vi "Webcam - Obstacle Box.vi"(0 "Image In":T1, 1 "Font, Size & Style":T2={"Desired Font (Application)"=enum."User-specified Font", "[User-specified Font]"={"Font Name"="", "Size"=50, "Strikeout?"=FALSE, "Italic?"=FALSE, "Underline?"=FALSE, "Outline?"=FALSE, "Shadow?"=FALSE, "Bold?"=TRUE, "Rotation Angle"=0.0}, "Horizontal Alignment"=0, "Vertical Alignment"=0} {"Vertical Alignment" items=["Bottom", "Top", "Baseline"]; "Horizontal Alignment" items=["Left", "Center", "Right"]; "[User-specified Font]"."Rotation Angle" format="%.2f"}, 2 "String":string="Obstacle", 3 "Text Color":u32(colorbox)=6618880, 5 "Left":i32, 7 "Top":i32, 9 "Right":i32, 11 "Bottom":i32, 12 "Color 1":u32(colorbox), 13 "Color 2":u32(colorbox)) -> (4 "Image Out":T1)   [LabVIEW 2011]
uses:
  <vilib>/vision/Image Controls.llb/IMAQ Image.ctl
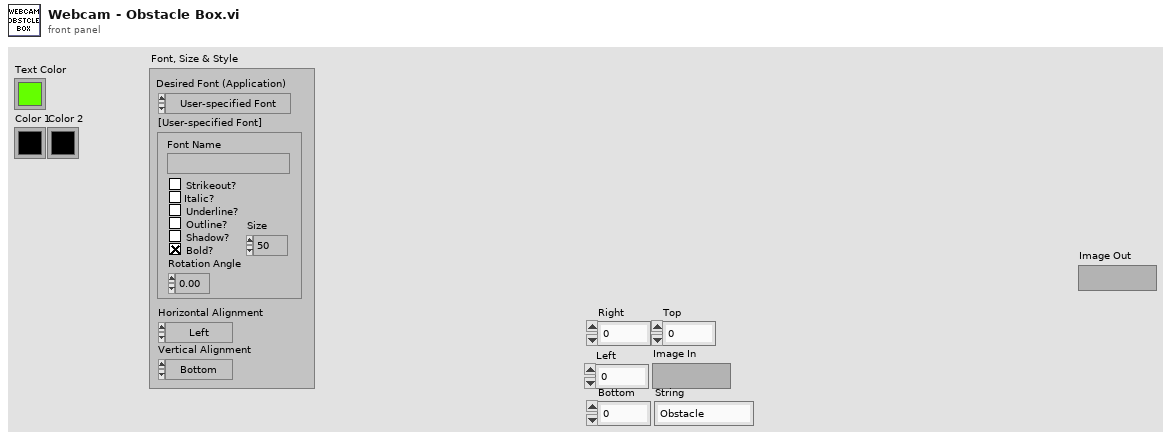
[diagram p1: front panel]
types:
  T1 = typedef "IMAQ Image.ctl" = refnum<image>
  T2 = cluster{"Desired Font (Application)":enum16{"User-specified Font", "Application Font", "System Font", "Dialog Font"}, "[User-specified Font]":cluster{"Font Name":string, "Size":i16, "Strikeout?":bool, "Italic?":bool, "Underline?":bool, "Outline?":bool, "Shadow?":bool, "Bold?":bool, "Rotation Angle":dbl}, "Horizontal Alignment":i16, "Vertical Alignment":i16}
  T3 = cluster{"Left":i32, "Top":i32, "Right":i32, "Bottom":i32}
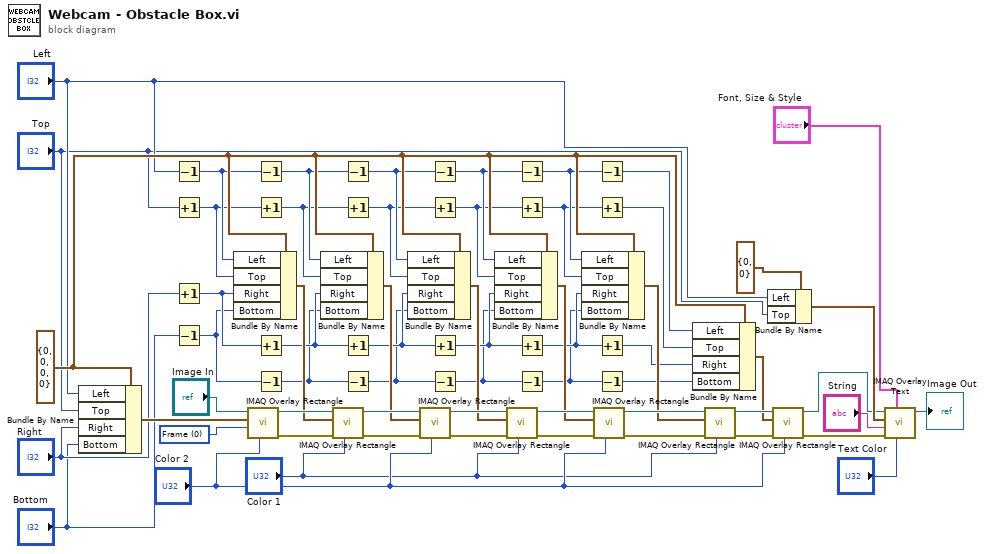
[diagram p0: block diagram]
diagram:
  w38 = T3 {"Left"=0, "Top"=0, "Right"=0, "Bottom"=0} ("input cluster")
  w60 = u32 0 items=["Frame", "Fill", "Highlight"] ("Drawing Mode (Frame)")
  n1 = Bundle By Name(cluster=w38, "Left"="Left", "Top"="Top", "Right"="Right", "Bottom"="Bottom") -> (w57:T3)
  n2 = Decrement(x="Left") -> (x-1=w25:i32)
  n3 = Increment(x="Top") -> (x+1=w24:i32)
  n4 = Increment(x="Right") -> (x+1=w23:i32)
  n5 = Decrement(x="Bottom") -> (x-1=w22:i32)
  n6 = Bundle By Name(cluster=w38, "Left"=w25, "Top"=w24, "Right"=w23, "Bottom"=w22) -> (w37:T3)
  n7 = call "IMAQ Overlay Rectangle"("Color"="Color 2", "Drawing Mode (Frame)"=w60, "Rectangle"=w57, "Image"="Image In") -> ("error out"=w52:errorcluster, "Image Out"=w51:T1)  [unwired: 6 in]
  n8 = Decrement(x=w25) -> (x-1=w21:i32)
  n9 = Increment(x=w24) -> (x+1=w20:i32)
  n10 = Increment(x=w23) -> (x+1=w19:i32)
  n11 = Decrement(x=w22) -> (x-1=w18:i32)
  n12 = Bundle By Name(cluster=w38, "Left"=w21, "Top"=w20, "Right"=w19, "Bottom"=w18) -> (w36:T3)
  n13 = call "IMAQ Overlay Rectangle"("Color"="Color 1", "error in (no error)"=w52, "Rectangle"=w37, "Image"=w51) -> ("error out"=w50:errorcluster, "Image Out"=w49:T1)  [unwired: 6 in]
  n14 = Decrement(x=w21) -> (x-1=w17:i32)
  n15 = Increment(x=w20) -> (x+1=w16:i32)
  n16 = Increment(x=w19) -> (x+1=w15:i32)
  n17 = Decrement(x=w18) -> (x-1=w14:i32)
  n18 = Bundle By Name(cluster=w38, "Left"=w17, "Top"=w16, "Right"=w15, "Bottom"=w14) -> (w35:T3)
  n19 = call "IMAQ Overlay Rectangle"("Color"="Color 2", "error in (no error)"=w50, "Rectangle"=w36, "Image"=w49) -> ("error out"=w39:errorcluster, "Image Out"=w40:T1)  [unwired: 6 in]
  n20 = Decrement(x=w17) -> (x-1=w13:i32)
  n21 = Increment(x=w16) -> (x+1=w12:i32)
  n22 = Increment(x=w15) -> (x+1=w11:i32)
  n23 = Decrement(x=w14) -> (x-1=w10:i32)
  n24 = Bundle By Name(cluster=w38, "Left"=w13, "Top"=w12, "Right"=w11, "Bottom"=w10) -> (w34:T3)
  n25 = call "IMAQ Overlay Rectangle"("Color"="Color 1", "error in (no error)"=w39, "Rectangle"=w35, "Image"=w40) -> ("error out"=w48:errorcluster, "Image Out"=w47:T1)  [unwired: 6 in]
  n26 = Decrement(x=w13) -> (x-1=w9:i32)
  n27 = Increment(x=w12) -> (x+1=w8:i32)
  n28 = Increment(x=w11) -> (x+1=w7:i32)
  n29 = Decrement(x=w10) -> (x-1=w6:i32)
  n30 = Bundle By Name(cluster=w38, "Left"=w9, "Top"=w8, "Right"=w7, "Bottom"=w6) -> (w33:T3)
  n31 = call "IMAQ Overlay Rectangle"("Color"="Color 2", "error in (no error)"=w48, "Rectangle"=w34, "Image"=w47) -> ("error out"=w46:errorcluster, "Image Out"=w45:T1)  [unwired: 6 in]
  n32 = Decrement(x=w9) -> (x-1=w31:i32)
  n33 = Increment(x=w8) -> (x+1=w30:i32)
  n34 = Increment(x=w7) -> (x+1=w29:i32)
  n35 = Decrement(x=w6) -> (x-1=w28:i32)
  n36 = Bundle By Name(cluster=w38, "Left"=w31, "Top"=w30, "Right"=w29, "Bottom"=w28) -> (w32:T3)
  n37 = call "IMAQ Overlay Rectangle"("Color"="Color 1", "error in (no error)"=w46, "Rectangle"=w33, "Image"=w45) -> ("error out"=w44:errorcluster, "Image Out"=w43:T1)  [unwired: 6 in]
  n38 = Bundle By Name(cluster=cluster{"Left":i32, "Top":i32} {"Left"=0, "Top"=0} ("input cluster"), "Left"="Left", "Top"="Top") -> (w55:cluster{"Left":i32, "Top":i32})
  n39 = call "IMAQ Overlay Rectangle"("Color"="Color 2", "error in (no error)"=w44, "Rectangle"=w32, "Image"=w43) -> ("error out"=w41:errorcluster, "Image Out"=w42:T1)  [unwired: 6 in]
  n40 = call "IMAQ Overlay Text"("Text Color (black)"="Text Color", "Font, Size & Style"="Font, Size & Style", "error in (no error)"=w41, "String"="String", "Origin"=w55, "Image"=w42) -> ("Image Out"=→"Image Out":T1)  [unwired: 4 in, 1 out]
